vi "3DMotion.vi"(6 "phi":dbl, 9 "psi":dbl, 10 "th":dbl, 11 "SceneObject in":refnum<vi>) -> ()   [LabVIEW 2011]
uses:
  <vilib>/picture/3D Picture Control/NI_3D Picture Control.lvlib
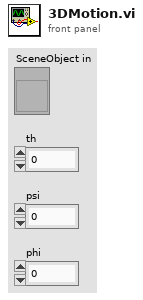
[diagram p1: front panel]
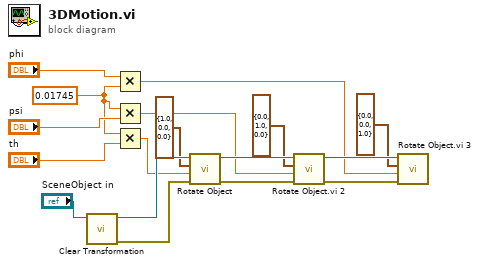
[diagram p0: block diagram]
diagram:
  w1 = 0.01745 ("x")
  n1 = call <vilib>:"Clear Transformation.vi"("Object Refnum In"="SceneObject in") -> ("error out"=w12:errorcluster, "Object Refnum Out"=w13:refnum<vi>)  [unwired: 9 in]
  n2 = Multiply(x="phi", y=w1) -> (x*y=w4:dbl)
  n3 = Multiply(x=w1, y="psi") -> (x*y=w3:dbl)
  n4 = Multiply(x=w1, y="th") -> (x*y=w2:dbl)
  n5 = call <vilib>:"Rotate Object.vi"("error in (no error)"=w12, "Angle"=w2, "Axis"=cluster{"X":sgl, "Y":sgl, "Z":sgl} {"X"=1.0, "Y"=0.0, "Z"=0.0}, "Scene.Object In"=w13) -> ("error out"=w8:errorcluster, "Scene.Object Out"=w11:refnum<vi>)  [unwired: 6 in]
  n6 = call "Rotate Object.vi 2"("error in (no error)"=w8, "Angle"=w3, "Axis"=cluster{"X":sgl, "Y":sgl, "Z":sgl} {"X"=0.0, "Y"=1.0, "Z"=0.0}, "Scene.Object In"=w11) -> ("error out"=w9:errorcluster, "Scene.Object Out"=w10:refnum<vi>)  [unwired: 6 in]
  n7 = call "Rotate Object.vi 3"("error in (no error)"=w9, "Angle"=w4, "Axis"=cluster{"X":sgl, "Y":sgl, "Z":sgl} {"X"=0.0, "Y"=0.0, "Z"=1.0}, "Scene.Object In"=w10) -> ()  [unwired: 6 in, 2 out]
